vi "Zero Padding.vi"(11 "Array in":cdb[](array[numeric])) -> (3 "Array out":cdb[](array[numeric]))   [LabVIEW 2014]
doc: "Pads begining and end of symbols up to size N (for N-Point IFFT)"
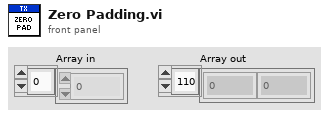
[diagram p1: front panel]
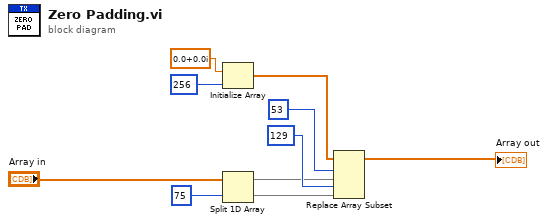
[diagram p0: block diagram]
diagram:
  n1 = Initialize Array "Initialize Array"(cdb 0.0+0.0i ("element"), 256 ("dimension size")) -> (w6:cdb[])
  n2 = Split 1D Array(array="Array in", index=75) -> (first subarray=w2:cdb[], second subarray=w1:cdb[])
  n3 = Replace Array Subset "Replace Array Subset"(array=w6, new element #1=w2, index #1=53 ("index"), new element #2=w1, index #2=129 ("index")) -> (→"Array out":cdb[])
